vi "写入-数据库操作.lvclass.vi"(8 "error in (no error)":errorcluster caption="错误输入（无错误）", 10 "数据库操作.lvclass":refnum<class "数据库操作.lvclass">, 11 "PC总客户端输入":refnum<class "PC总客户端.lvclass">) -> (0 "error out":errorcluster caption="错误输出", 3 "PC总客户端输出":refnum<class "PC总客户端.lvclass">)   [LabVIEW 2013, in "PC总客户端.lvclass"]
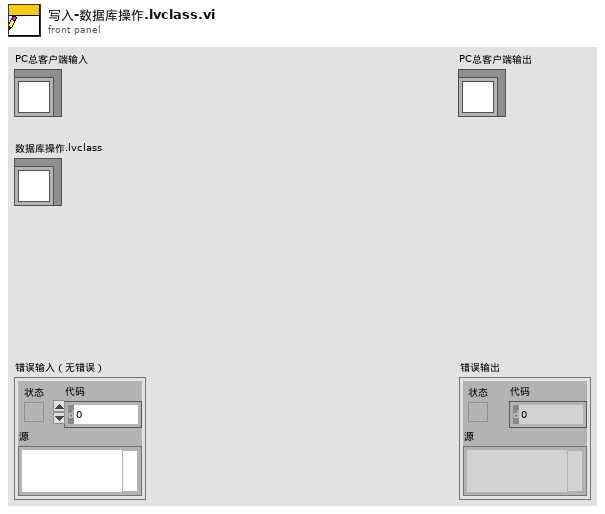
[diagram p1: front panel]
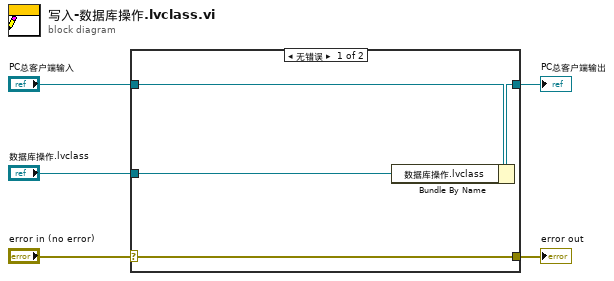
[diagram p0: block diagram]
diagram:
  n1 = case shown="无错误" "error in (no error)" {
    selector: "error in (no error)" -> [w9 w10]
    tunnel: [w9 w10] -> w4
    tunnel: [w7 w11] -> w2
    tunnel: "PC总客户端输入" -> [w8 w11]
    tunnel: "数据库操作.lvclass" -> [w6 _]
    frame No Error {
      n2 = Bundle By Name(cluster=w8, "数据库操作.lvclass"=w6) -> (w7:refnum<class "PC总客户端.lvclass">)
    }
    frame Error {
    }
  }
  "error out" <- w4
  "PC总客户端输出" <- w2
